vi "Relay Status.vi"(8 "error in (no error)":errorcluster, 10 "Relay (1:1)":u16(ring)=1 items=["1"=1, "2"=2], 11 "VISA resource name":refnum<visa-resource-name>) -> (0 "error out":errorcluster, 2 "Relay On?":bool, 3 "VISA resource name out":refnum<visa-resource-name>)   [LabVIEW 2021, in "Lake Shore 336.lvlib"]
doc: "This VI returns the Relay status."
uses:
  <instrlib>/Lake Shore 336/Lake Shore 336.lvlib
  Instance           1 20Saved   Relay Status .vi
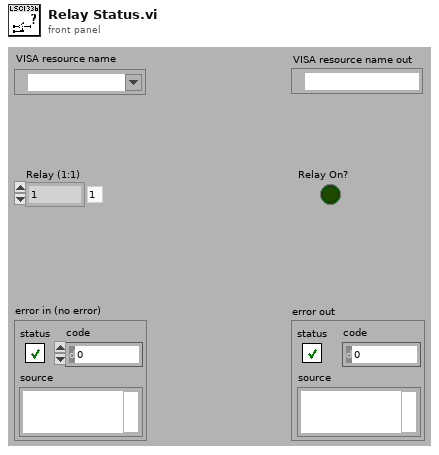
[diagram p1: front panel]
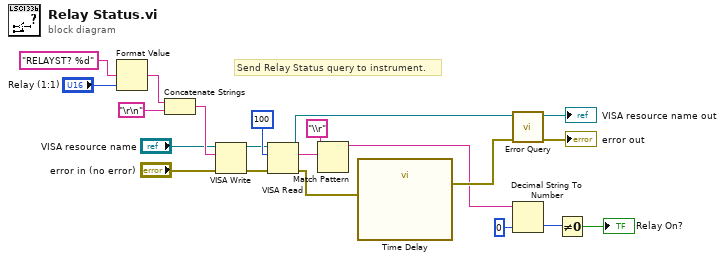
[diagram p0: block diagram]
diagram:
  # "Send Relay Status query to instrument."
  n1 = Format Value(format string="RELAYST? %d", value (0)="Relay (1:1)") -> (output string=w1:string)  [unwired: 1 in]
  n2 = Concatenate Strings(w1, "\r\n") -> (w11:string)
  n3 = VISA Write(VISA resource name="VISA resource name", write buffer=w11, error in (no error)="error in (no error)") -> (VISA resource name out=w15:refnum<visa-resource-name>, error out=w14:errorcluster)  [unwired: 1 out]
  n4 = VISA Read(VISA resource name=w15, byte count=100, error in (no error)=w14) -> (VISA resource name out=w9:refnum<visa-resource-name>, read buffer=w17:string, error out=w13:errorcluster)  [unwired: 1 out]
  n5 = Match Pattern(string=w17, regular expression="\\r") -> (before substring=w8:string)  [unwired: 1 in, 3 out]
  n6 = call "Time Delay"("error in (no error)"=w13) -> ("error out"=w10:errorcluster)  [unwired: 10 in]
  n7 = call <instrlib>:"Error Query.vi"("error in (no error)"=w10, "VISA resource name"=w9) -> ("error out"=→"error out":errorcluster, "VISA resource name out"=→"VISA resource name out":refnum<visa-resource-name>)  [unwired: 7 in, 1 out]
  n8 = Decimal String To Number(string=w8, default (0L)=u16 0) -> (number=w5:u16)  [unwired: 1 in, 1 out]
  n9 = Not Equal To 0?(x=w5) -> (x != 0?=→"Relay On?":bool)
